vi "Orifice_Z.vi"(7 "nu":dbl, 8 "rho":dbl, 9 "Ho":dbl, 10 "Do/2":dbl, 11 "Omega":dbl) -> (3 "Zo":cdb)   [LabVIEW 2022 SP3]
uses:
  <vilib>/Analysis/8numeric.llb/Numeric Integration.vi
  <vilib>/Analysis/8numeric.llb/1D Numeric Integration.vi
  <vilib>/Analysis/1siggen.llb/Ramp Pattern.vi
  <vilib>/Analysis/1siggen.llb/Ramp Pattern by Delta.vi
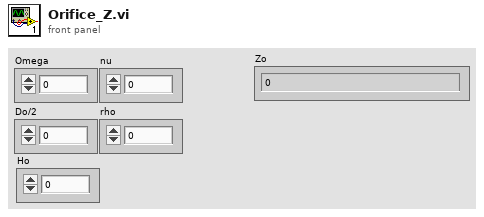
[diagram p1: front panel]
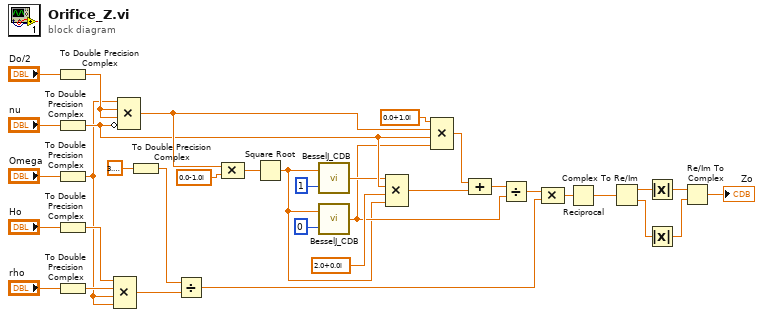
[diagram p0: block diagram]
diagram:
  n1 = To Double Precision Complex(1:"Do/2") -> (0:w27:cdb)
  n2 = To Double Precision Complex(1:"nu") -> (0:w20:cdb)
  n3 = To Double Precision Complex(1:"Omega") -> (0:w13:cdb)
  n4 = To Double Precision Complex(1:"Ho") -> (0:w15:cdb)
  n5 = To Double Precision Complex(1:"rho") -> (0:w14:cdb)
  n6 = Compound Arithmetic op=MULTIPLY(w15, w14, w13, w13) -> (w12:cdb)
  n7 = Compound Arithmetic op=MULTIPLY(w13, w27, w27, invert w20) -> (w25:cdb)
  n8 = To Double Precision Complex(1:3.141592653589793) -> (0:w11:cdb)
  n9 = Divide(x=w11, y=w12) -> (x/y=w9:cdb)
  n10 = Compound Arithmetic op=MULTIPLY(w25, cdb 0.0-1.0i ("value")) -> (w23:cdb)
  n11 = Square Root(x=w23) -> (sqrt(x)=w7:cdb)
  n12 = call "BesselJ_CDB.vi"("n"=1 ("order"), "a+bi"=w7) -> ("Jn(a+bi)"=w19:cdb)
  n13 = call "BesselJ_CDB.vi"("n"=0 ("order"), "a+bi"=w7) -> ("Jn(a+bi)"=w16:cdb)
  n14 = Compound Arithmetic op=MULTIPLY(w19, w20, cdb 2.0+0.0i ("value"), w7) -> (w18:cdb)
  n15 = Compound Arithmetic op=MULTIPLY(cdb 0.0+1.0i ("value"), w25, w20, w16) -> (w22:cdb)
  n16 = Compound Arithmetic op=ADD(w22, w18) -> (w17:cdb)
  n17 = Divide(x=w17, y=w16) -> (x/y=w10:cdb)
  n18 = Compound Arithmetic op=MULTIPLY(w10, w9) -> (w8:cdb)
  n19 = Reciprocal(x=w8) -> (1/x=w6:cdb)
  n20 = Complex To Re/Im(x + iy=w6) -> (x=w3:dbl, y=w5:dbl)
  n21 = Absolute Value(x=w3) -> (abs(x)=w1:dbl)
  n22 = Absolute Value(x=w5) -> (abs(x)=w2:dbl)
  n23 = Re/Im To Complex(1:w2, 2:w1) -> (0:→"Zo":cdb)
